vi "New.vi"(8 "error in (no error)":errorcluster, 11 "PrettyPrint?":bool) -> (0 "error out":errorcluster, 3 "BlueJSONTextSerializer out":refnum<class "BlueJSONTextSerializer.lvclass">)   [LabVIEW 2019, in "BlueJSONTextSerializer.lvlib" / "BlueJSONTextSerializer.lvclass"]
uses:
  BlueJSONTextSerializer.lvclass
  BlueJSONTextSerializer.lvclass/BlueJSONTextSerializer.ctl
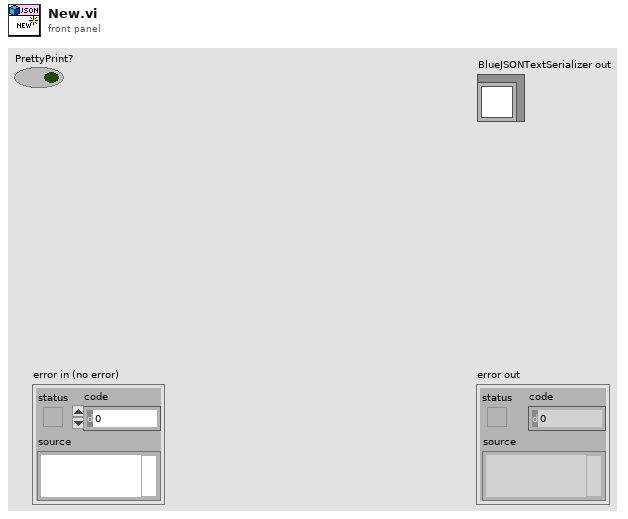
[diagram p1: front panel]
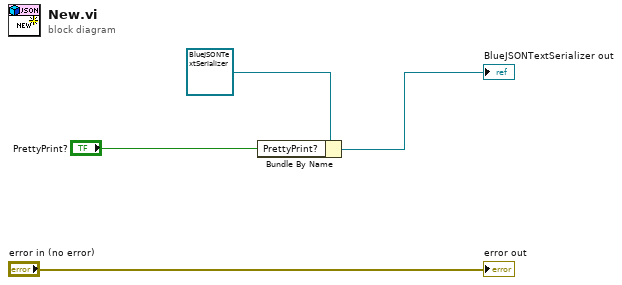
[diagram p0: block diagram]
diagram:
  n1 = Bundle By Name(cluster=refnum<class "BlueJSONTextSerializer.lvclass"> refnum ("BlueJSONTextSerializer out"), "PrettyPrint?"="PrettyPrint?") -> (→"BlueJSONTextSerializer out":refnum<class "BlueJSONTextSerializer.lvclass">)
  "error out" <- "error in (no error)"
